vi "PYTHON VI Tree__ogtk.vi"() -> ()   [LabVIEW 2014]
uses:
  <userlib>/_OpenG.lib/labpython/labpython.llb/PYTHON Session Refnum__ogtk.ctl
panel:
  out "Python Session":T1
  # "PYTHON VI Tree.vi\n\nAn overview of all user functions from the Python VI Library\n\nCopyright (C) 2002 Rolf Kalbermatter rolf.kalbermatter@citeng.com\nCopyright (C) 2002 James Kring jim@jimkring.com\n\nPlease visit http://www.OpenG.org to learn about the\nOpen Source LabVIEW software movement.\n\nThis library is free software; you can redistribute it and/or\nmodify it under the terms of the GNU Lesser General Public\nLicense as published by the Free Software Foundation; either\nversion 2.1 of the License, or (at your option) any later version.\nThis library is distributed in the hope that it will be useful,\nbut WITHOUT ANY WARRANTY; without even the implied warranty of\nMERCHANTABILITY or FITNESS FOR A PARTICULAR PURPOSE. See the GNU\nLesser General Public License for more details.\nYou should have received a copy of the GNU Lesser General Public\nLicense along with this library; if not, write to the Free Software\nFoundation, Inc., 59 Temple Place, Suite 330, Boston, MA 02111-1307 USA"
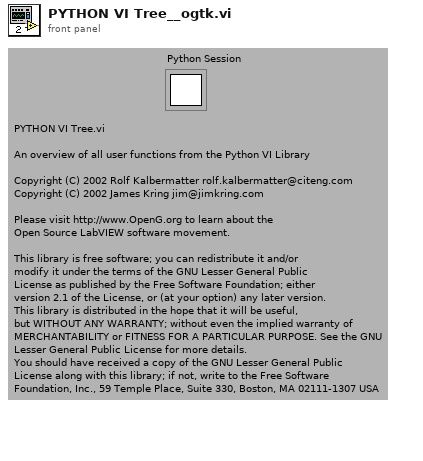
[diagram p1: front panel]
types:
  T1 = typedef "PYTHON Session Refnum__ogtk.ctl" = refnum<k1>
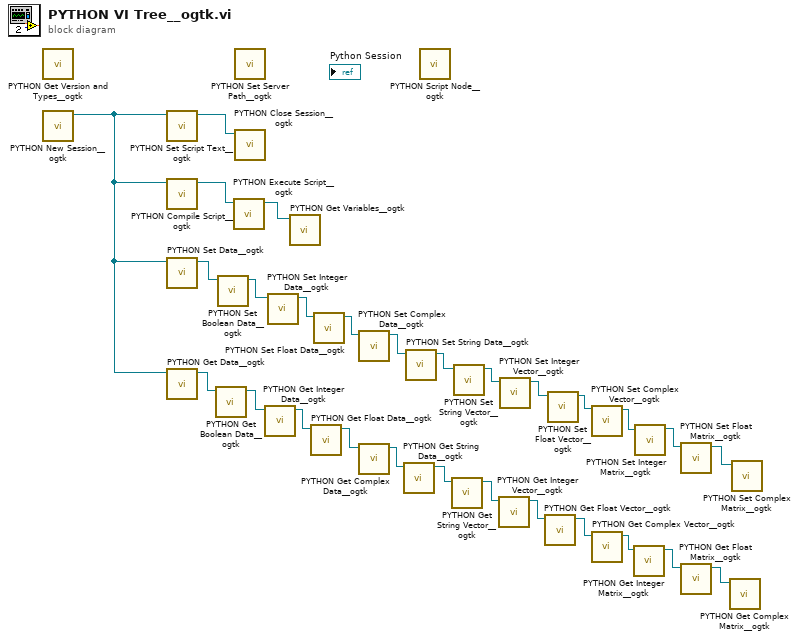
[diagram p0: block diagram]
diagram:
  n1 = call <userlib>:"PYTHON Get Version and Types__ogtk.vi"() -> ()  [unwired: 5 in, 3 out]
  n2 = call <userlib>:"PYTHON New Session__ogtk.vi"() -> ("Python Session"=w22:T1)  [unwired: 6 in, 1 out]
  n3 = call <userlib>:"PYTHON Set Script Text__ogtk.vi"("Python Session in"=w22) -> ("Python Session out"=w28:T1)  [unwired: 5 in, 1 out]
  n4 = call <userlib>:"PYTHON Compile Script__ogtk.vi"("Python Session in"=w22) -> ("Python Session out"=w23:T1)  [unwired: 5 in, 1 out]
  n5 = call-poly <userlib>:"PYTHON Set Data__ogtk.vi"("Python Session in"=w22) -> ("Python Session out"=w27:T1)  [unwired: 5 in, 1 out]
  n6 = call-poly <userlib>:"PYTHON Get Data__ogtk.vi"("Python Session in"=w22) -> ("Python Session out"=w17:T1)  [unwired: 4 in, 2 out]
  n7 = call <userlib>:"PYTHON Get Boolean Data__ogtk.vi"("Python Session in"=w17) -> ("Python Session out"=w16:T1)  [unwired: 4 in, 2 out]
  n8 = call <userlib>:"PYTHON Set Boolean Data__ogtk.vi"("Python Session in"=w27) -> ("Python Session out"=w15:T1)  [unwired: 5 in, 1 out]
  n9 = call <userlib>:"PYTHON Execute Script__ogtk.vi"("Python Session in"=w23) -> ("Python Session out"=w18:T1)  [unwired: 5 in, 1 out]
  n10 = call <userlib>:"PYTHON Set Server Path__ogtk.vi"() -> ()  [unwired: 7 in, 1 out]
  n11 = call <userlib>:"PYTHON Close Session__ogtk.vi"("Python Session in"=w28) -> ()  [unwired: 6 in, 1 out]
  n12 = call <userlib>:"PYTHON Get Integer Data__ogtk.vi"("Python Session in"=w16) -> ("Python Session out"=w21:T1)  [unwired: 4 in, 2 out]
  n13 = call <userlib>:"PYTHON Set Integer Data__ogtk.vi"("Python Session in"=w15) -> ("Python Session out"=w26:T1)  [unwired: 5 in, 1 out]
  n14 = call <userlib>:"PYTHON Get Variables__ogtk.vi"("Python Session in"=w18) -> ()  [unwired: 3 in, 4 out]
  n15 = call <userlib>:"PYTHON Get Float Data__ogtk.vi"("Python Session in"=w21) -> ("Python Session out"=w20:T1)  [unwired: 4 in, 2 out]
  n16 = call <userlib>:"PYTHON Set Float Data__ogtk.vi"("Python Session in"=w26) -> ("Python Session out"=w25:T1)  [unwired: 5 in, 1 out]
  n17 = call <userlib>:"PYTHON Set Complex Data__ogtk.vi"("Python Session in"=w25) -> ("Python Session out"=w24:T1)  [unwired: 5 in, 1 out]
  n18 = call <userlib>:"PYTHON Get Complex Data__ogtk.vi"("Python Session in"=w20) -> ("Python Session out"=w19:T1)  [unwired: 4 in, 2 out]
  n19 = call <userlib>:"PYTHON Get String Data__ogtk.vi"("Python Session in"=w19) -> ("Python Session out"=w4:T1)  [unwired: 4 in, 2 out]
  n20 = call <userlib>:"PYTHON Set String Data__ogtk.vi"("Python Session in"=w24) -> ("Python Session out"=w2:T1)  [unwired: 5 in, 1 out]
  n21 = call <userlib>:"PYTHON Script Node__ogtk.vi"() -> ()  [unwired: 1 in]
  n22 = call <userlib>:"PYTHON Get String Vector__ogtk.vi"("Python Session in"=w4) -> ("Python Session out"=w3:T1)  [unwired: 4 in, 2 out]
  n23 = call <userlib>:"PYTHON Set String Vector__ogtk.vi"("Python Session in"=w2) -> ("Python Session out"=w1:T1)  [unwired: 5 in, 1 out]
  n24 = call <userlib>:"PYTHON Get Integer Vector__ogtk.vi"("Python Session in"=w3) -> ("Python Session out"=w14:T1)  [unwired: 4 in, 2 out]
  n25 = call <userlib>:"PYTHON Set Integer Vector__ogtk.vi"("Python Session in"=w1) -> ("Python Session out"=w9:T1)  [unwired: 5 in, 1 out]
  n26 = call <userlib>:"PYTHON Get Float Vector__ogtk.vi"("Python Session in"=w14) -> ("Python Session out"=w13:T1)  [unwired: 4 in, 2 out]
  n27 = call <userlib>:"PYTHON Set Float Vector__ogtk.vi"("Python Session in"=w9) -> ("Python Session out"=w8:T1)  [unwired: 5 in, 1 out]
  n28 = call <userlib>:"PYTHON Set Complex Vector__ogtk.vi"("Python Session in"=w8) -> ("Python Session out"=w7:T1)  [unwired: 5 in, 1 out]
  n29 = call <userlib>:"PYTHON Get Complex Vector__ogtk.vi"("Python Session in"=w13) -> ("Python Session out"=w12:T1)  [unwired: 4 in, 2 out]
  n30 = call <userlib>:"PYTHON Get Integer Matrix__ogtk.vi"("Python Session in"=w12) -> ("Python Session out"=w11:T1)  [unwired: 4 in, 2 out]
  n31 = call <userlib>:"PYTHON Set Integer Matrix__ogtk.vi"("Python Session in"=w7) -> ("Python Session out"=w6:T1)  [unwired: 5 in, 1 out]
  n32 = call <userlib>:"PYTHON Set Float Matrix__ogtk.vi"("Python Session in"=w6) -> ("Python Session out"=w5:T1)  [unwired: 5 in, 1 out]
  n33 = call <userlib>:"PYTHON Get Float Matrix__ogtk.vi"("Python Session in"=w11) -> ("Python Session out"=w10:T1)  [unwired: 4 in, 2 out]
  n34 = call <userlib>:"PYTHON Get Complex Matrix__ogtk.vi"("Python Session in"=w10) -> ()  [unwired: 4 in, 3 out]
  n35 = call <userlib>:"PYTHON Set Complex Matrix__ogtk.vi"("Python Session in"=w5) -> ()  [unwired: 5 in, 2 out]
